vi "Lab 6.vi"() -> ()   [LabVIEW 2010]
uses:
  <vilib>/Utility/file.llb/Write To Spreadsheet File (I64).vi
panel:
  in  "Data file path ending":string=".dat"
  in  "Auto Save Data":bool=TRUE
  in  "time format string (%c)":string="%Y-%m-%d %H-%M.%S"
  out "date/time string":string="2012-02-20 12-35.08"
  out "Previous acquisition":u16[](graph)
  out "ErrMsg":string="No error has occurred"
  out "ErrCode":i32
  out "Current acquisition":u16[](graph)
  in  "Range":i32(ring)=1 items=["Not Programmable"=0, "+- 20 V"=27, "+- 10 V"=1, "+- 5 V"=2, "+- 4 V"=28, "+- 2.5 V"=3, "+- 2 V"=29, "+- 1.67 V"=4, "+- 1.25 V"=5, "+- 1 V"=6, "+- .625 V"=7, "+- .5 V"=8, "+- .25 V"=30, "+- .2 V"=31, "+- .1 V"=9, "+- .05 V"=10, "+- .01 V"=11, "+- .005 V"=12, "0 - 10 V"=13, "0 - 5 V"=14, "0 - 4 V"=36, "0 - 2.5 V"=15, "0 - 2 V"=16, "0 - 1.67 V"=17, "0 - 1.25 V"=18, "0 - 1 V"=19, "0 - .5 V"=32, "0 - .25 V"=33, "0 - .2 V"=34, "0 - .1 V"=20, "0 - .02 V"=35, "0 - .01 V"=21, "4 - 20 mA"=22, "2 - 10 mA"=23, "1 - 5 mA"=24, ".5 - 2.5 mA"=25, "0 - 20 mA"=26]
  in  "InterChannel Delay":sgl=-1.0 format="%.2f"
  in  "Options":i32
  in  "Rate":i32=3000
  in  "Count":i32=1000
  in  "HighChan":i32
  in  "LowChan":i32
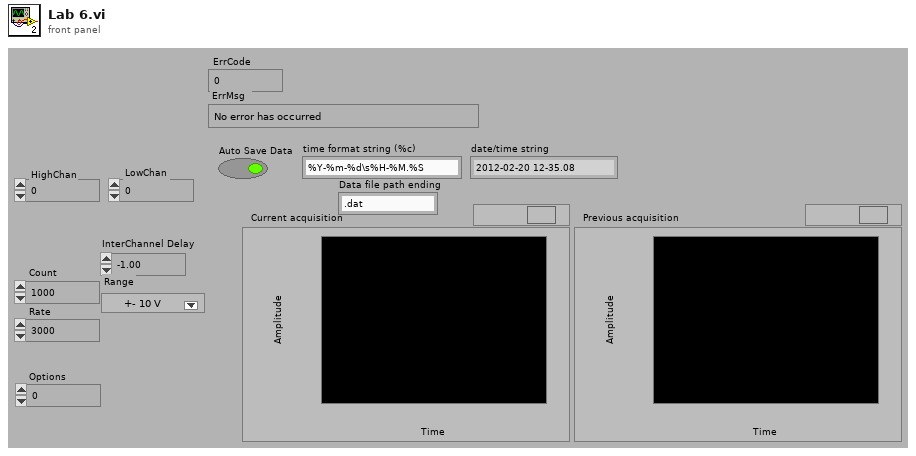
[diagram p1: front panel]
types:
  T1 = typedef "imagedata.ctl" = cluster{"image type":i32, "image depth":i32, "image":u8[], "mask":u8[], "colors":u32[], "Rectangle":cluster{"left":i16, "top":i16, "right":i16, "bottom":i16}}
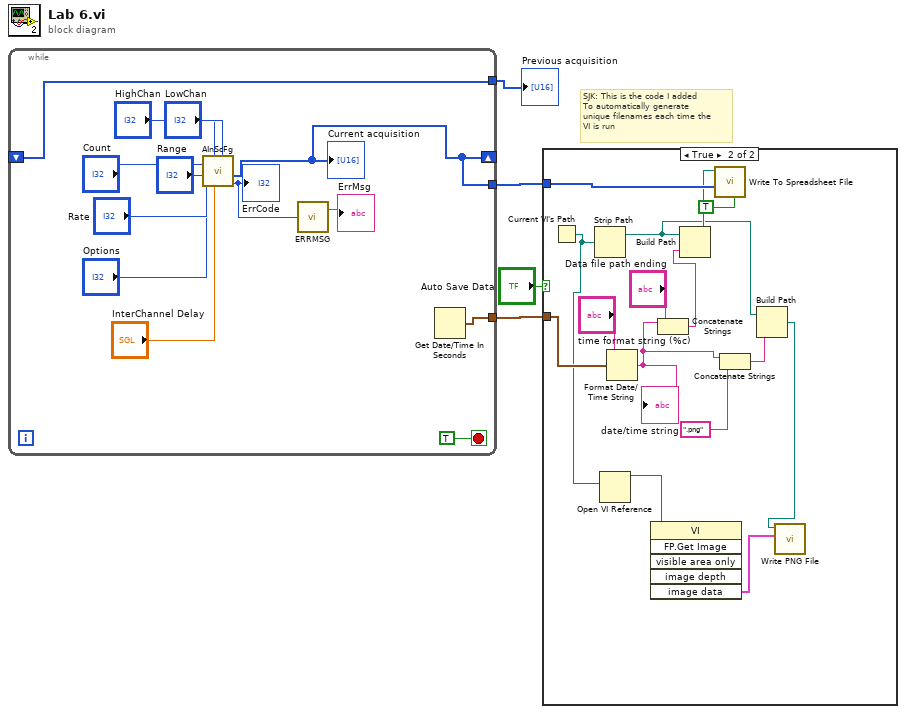
[diagram p0: block diagram]
diagram:
  # "SJK: This is the code I added\nTo automatically generate \nunique filenames each time the\nVI is run"
  n1 = while {
    shift-right: [w6] -> _
    shift-left: _ -> [w7]
    tunnel: [w7] -> w4
    tunnel: [w6] -> w3
    tunnel: [w5] -> w2
    stop <- TRUE stop-if-true
    n2 = call <menus>:"AInScFg.VI"("LowChan"="LowChan", "InterChannel Delay"="InterChannel Delay", "HighChan"="HighChan", "Options"="Options", "Range"="Range", "Rate"="Rate", "Count"="Count") -> ("ErrCode"=w10:i32, "ADData"=w6:u16[])  [unwired: 1 in, 1 out]
    "Current acquisition" <- w6
    "ErrCode" <- w10
    n3 = call <menus>:"ERRMSG.VI"("ErrCode"=w10) -> ("ErrMsg"=→"ErrMsg":string)  [unwired: 1 out]
    n4 = Get Date/Time In Seconds() -> (seconds since 1Jan1904=w5:timestamp)
  }
  "Previous acquisition" <- w4
  n5 = case shown="True" "Auto Save Data" {
    tunnel: w3 -> [_ w32]
    tunnel: w2 -> [_ w31]
    frame False {
    }
    frame True {
      n6 = Current VI's Path() -> (path=w23:path)
      n7 = Strip Path(path=w23) -> (stripped path=w22:path)  [unwired: 1 out]
      n8 = Open VI Reference(vi path=w23) -> (vi reference=w24:refnum<vi>)  [unwired: 5 in, 1 out]
      n9 = Format Date/Time String(time format string (%c)="time format string (%c)", seconds (now)=w31) -> (date/time string=w21:string)  [unwired: 1 in]
      "date/time string" <- w21
      n10 = invoke class="VI" method="FP.Get Image"(reference=w24) -> ("image data"=w25:T1)  [unwired: 5 in, 5 out]
      n11 = Concatenate Strings(w21, "Data file path ending") -> (w28:string)
      n12 = Build Path(base path=w22, name or relative path=w28) -> (appended path=w27:path)
      n13 = call-poly <vilib>:"Write To Spreadsheet File.vi"("transpose? (no:F)"=TRUE, "1D data"=w32, "file path (dialog if empty)"=w27) -> ()  [unwired: 5 in, 1 out]
      n14 = Concatenate Strings(w21, ".png" ("string")) -> (w19:string)
      n15 = Build Path(base path=w22, name or relative path=w19) -> (appended path=w18:path)
      n16 = call <vilib>:"Write PNG File.vi"("image data"=w25, "path to PNG file"=w18) -> ()  [unwired: 8 in, 2 out]
    }
  }
